vi "Detect Devices.vi"(8 "error in (no error)":errorcluster, 11 "VISA resource name":refnum<visa-resource-name>) -> (0 "error out":errorcluster, 1 "Axis Counts by Device":i32[][](array[numeric]), 2 "Connected Devices and Axes":string[](array[string]), 3 "VISA resource name out":refnum<visa-resource-name>)   [LabVIEW 2021, in "Zaber A Series.lvlib"]
doc: "Polls the connected devices and returns an array of the Connected Devices and Axes. Elements of the array can be used as an input for the Device and Axis input of other VIs in this library, for example through a dropdown list.\n\nThis VI requires that the Initialize VI has been called with the same serial port."
uses:
  Zaber A Series.lvlib
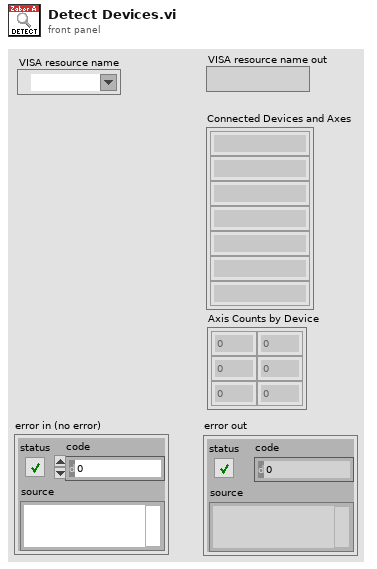
[diagram p1: front panel]
types:
  T1 = cluster{"Device":string, "Axis":string, "Reply Flag":string, "Status":string, "Warning Flags":string, "Data":string}[]
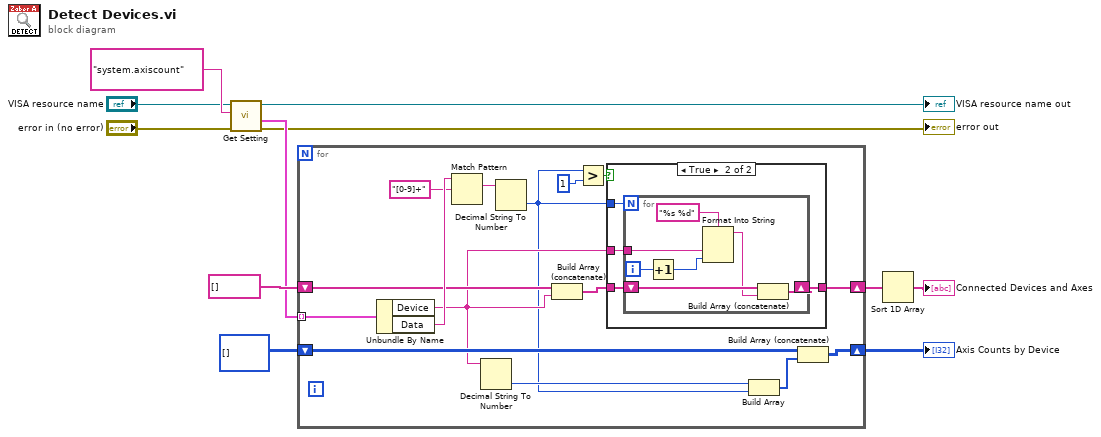
[diagram p0: block diagram]
diagram:
  n1 = call "Get Setting.vi"("error in (no error)"="error in (no error)", "Setting"="system.axiscount" ("Common Settings"), "VISA resource name"="VISA resource name") -> ("error out"=→"error out":errorcluster, "Response Bundle Array"=w5:T1, "VISA resource name out"=→"VISA resource name out":refnum<visa-resource-name>)  [unwired: 3 in, 3 out]
  n2 = for {
    tunnel: w5 -> [w12] mode=indexing
    shift-right: [w19] -> w9
    shift-left: string[] [] -> [w18]
    shift-right: [w22] -> w3
    shift-left: i32[][] [] -> [w21]
    n3 = Unbundle By Name(w12) -> ("Device"=w17:string, "Data"=w26:string)
    n4 = Match Pattern(string=w26, regular expression="[0-9]+") -> (match substring=w24:string)  [unwired: 1 in, 3 out]
    n5 = Decimal String To Number(string=w17) -> (number=w23:i32)  [unwired: 2 in, 1 out]
    n6 = Decimal String To Number(string=w24) -> (number=w13:i32)  [unwired: 2 in, 1 out]
    n7 = Build Array (concatenate)(w18, w17) -> (w16:string[])
    n8 = Greater?(x=w13, y=1) -> (0:w15:bool)
    n9 = case shown="True" w15 {
      tunnel: w13 -> [_ w31]
      tunnel: w17 -> [_ w30]
      tunnel: w16 -> [w27 w29]
      tunnel: [w27 w28] -> w19
      frame False {
      }
      frame True {
        n10 = for {
          N: w31 -> [_]
          tunnel: w30 -> [w34]
          shift-right: [w36] -> w28
          shift-left: w29 -> [w37]
          i -> [w38]
          n11 = Increment(x=w38) -> (x+1=w33:i32)
          n12 = Format Into String(format string="%s %d", w34, w33) -> (resulting string=w32:string)  [unwired: 2 in, 1 out]
          n13 = Build Array (concatenate)(w37, w32) -> (w36:string[])
        }
      }
    }
    n14 = Build Array(w23, w13) -> (w20:i32[])
    n15 = Build Array (concatenate)(w21, w20) -> (w22:i32[][])
  }
  "Axis Counts by Device" <- w3
  n16 = Sort 1D Array(array=w9) -> (sorted array=→"Connected Devices and Axes":string[])
